vi "Read All Sensor Data.vi"(8 "error in (no error)":errorcluster, 11 "LS218 in":refnum<class "LS218.lvclass">) -> (0 "error out":errorcluster, 3 "LS218 out":refnum<class "LS218.lvclass">)   [LabVIEW 2015, in "LS218.lvlib" / "LS218.lvclass"]
uses:
  LS218.lvclass
  PV-Enum.ctl
  LS218.lvclass/LS218.ctl
  CSPP_Core/Classes/CS++ProcessVariables/PVConnection/PVConnection.lvclass/PVConnection.ctl
  CSPP_Core/Classes/CS++ProcessVariables/ProcessVariable/PV.lvclass/PV.ctl
  CSPP_Core/Classes/CS++ProcessVariables/ProcessVariable/Write Data.vi
  CSPP_Core/Classes/CS++ProcessVariables/ProcessVariable/Write Error.vi
  CSPP_Core/Classes/CS++ProcessVariables/ProcessVariable/Write status.vi
  CSPP_Core/Classes/CS++ProcessVariables/ProcessVariable/Write Quality.vi
  CSPP_Core/Classes/CS++ProcessVariables/ProcessVariable/Write Timestamp.vi
  CSPP_Core/Classes/CS++ProcessVariables/ProcessVariable/PV.lvclass
  <instrlib>/Lake Shore Cryotronics 218/Lake Shore Cryotronics 218.lvlib
  CSPP_Core/Classes/CS++ProcessVariables/PVConnection/PVConnection.lvclass
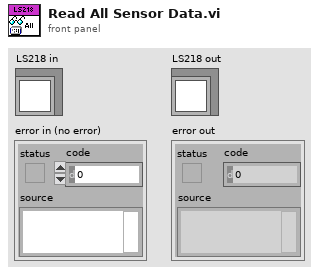
[diagram p1: front panel]
types:
  T1 = typedef "LS218.lvlib/LS218.lvclass/PV-Enum.ctl" = enum16{"T0", "T1", "T2", "T3", "T4", "T5", "T6", "T7", "Relay", "S0", "S1", "S2", "S3", "S4", "S5", "S6", "S7"}
  T2 = cluster{"Relay 1":bool, "Relay  2":bool, "Relay 3":bool, "Relay 4":bool, "Relay 5":bool, "Relay 6":bool, "Relay 7":bool, "Relay 8":bool}
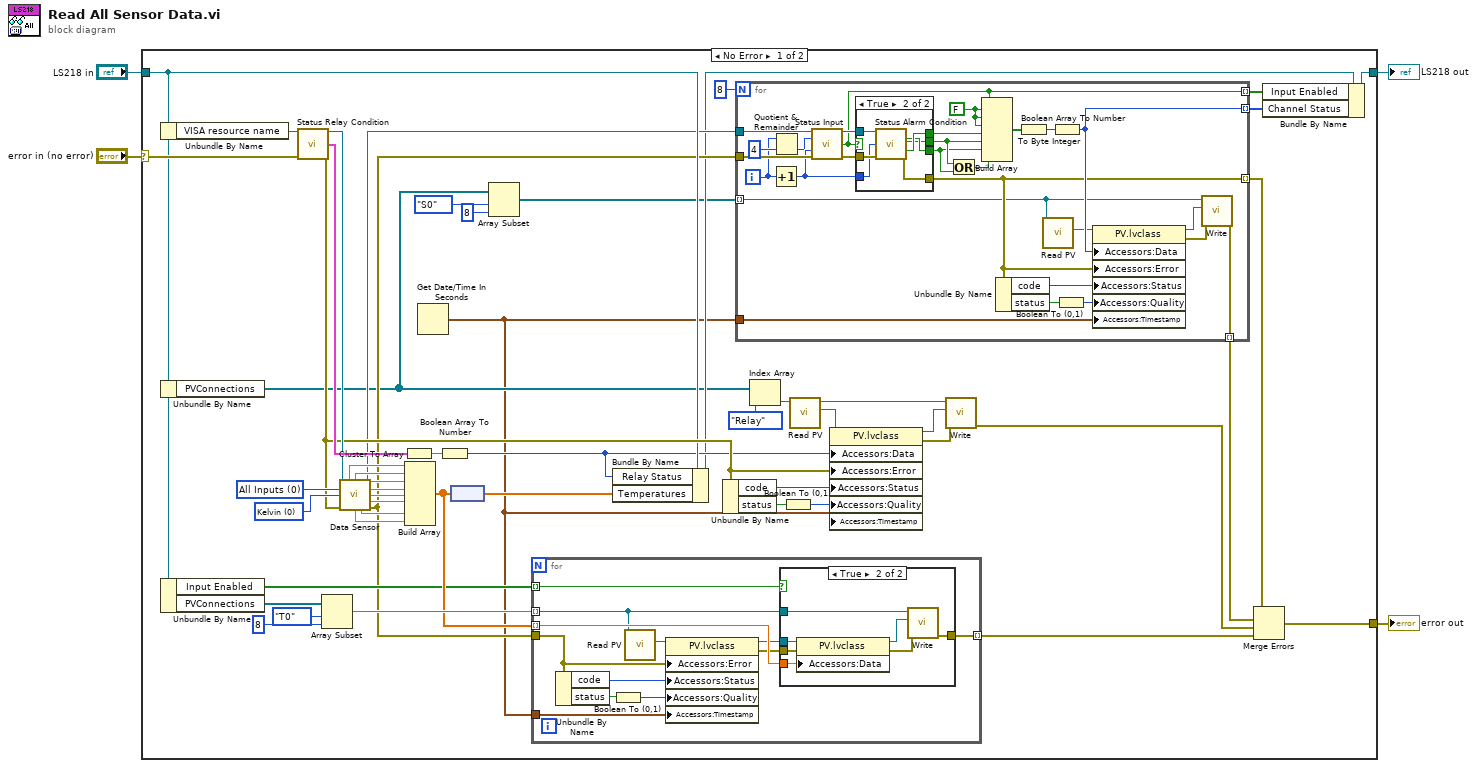
[diagram p0: block diagram]
diagram:
  n1 = case shown="No Error" "error in (no error)" {
    selector: "error in (no error)" -> [w28 w111]
    tunnel: [w40 w111] -> w3
    tunnel: [w17 w110] -> w1
    tunnel: "LS218 in" -> [w26 w110]
    frame No Error {
      w54 = u16 0 items=["All Inputs", "1", "2", "3", "4", "5", "6", "7", "8"] ("Input (0:All)")
      w55 = u16 0 items=["Kelvin", "Celsius", "Sensor Units", "Linear Data"] ("Data Source (0:Kelvin)")
      n2 = Unbundle By Name(w26) -> ("VISA resource name"=w30:refnum<visa-resource-name>)
      n3 = Unbundle By Name(w26) -> ("PVConnections"=w14:refnum<class "PVConnection.lvclass">[])
      n4 = Unbundle By Name(w26) -> ("Input Enabled"=w39:bool[], "PVConnections"=w44:refnum<class "PVConnection.lvclass">[])
      n5 = call <instrlib>:"Status Relay Condition.vi"("VISA resource name"=w30, "error in (no error)"=w28) -> ("VISA resource name out"=w29:refnum<visa-resource-name>, "Relay Status"=w37:T2, "error out"=w27:errorcluster)  [unwired: 11 in]
      n6 = Array Subset(array=w44, index=PV-Enum."T0" ("PV-Enum"), length=8) -> (w42:refnum<class "PVConnection.lvclass">[])
      n7 = call <instrlib>:"Data Sensor.vi"("VISA resource name"=w29, "Input (0:All)"=w54, "Data Source (0:Kelvin)"=w55, "error in (no error)"=w27) -> ("Input 1"=w53:dbl, "Input 2"=w52:dbl, "Input 3"=w51:dbl, "VISA resource name out"=w22:refnum<visa-resource-name>, "Input 4"=w50:dbl, "Input 5"=w49:dbl, "Input 6"=w48:dbl, "Input 8"=w46:dbl, "Input 7"=w47:dbl, "error out"=w21:errorcluster)  [unwired: 2 in]
      n8 = Cluster To Array(cluster=w37) -> (array=w38:bool[])
      n9 = Build Array(w53, w52, w51, w50, w49, w48, w47, w46) -> (w41:dbl[])
      n10 = Get Date/Time In Seconds() -> (seconds since 1Jan1904=w10:timestamp)
      n11 = Boolean Array To Number(Boolean array=w38) -> (number=w25:u32)
      n12 = node(w41) -> (w45:dbl[unit][])
      n13 = Array Subset(array=w14, index=PV-Enum."S0" ("PV-Enum"), length=8) -> (w11:refnum<class "PVConnection.lvclass">[])
      n14 = for {
        tunnel: w42 -> [w57] mode=indexing
        tunnel: w41 -> [w64] mode=indexing
        tunnel: w39 -> [w62] mode=indexing
        tunnel: w10 -> [w58]
        tunnel: w21 -> [w59]
        tunnel: [w60] -> w23 mode=indexing
        n15 = Unbundle By Name(w59) -> ("code"=w67:i32, "status"=w66:bool)
        n16 = Boolean To (0,1)(Boolean=w66) -> (0, 1=w65:i16)
        n17 = call "Read PV.vi"("PVConnection in"=w57) -> ("PV"=w56:refnum<class "PV.lvclass">)  [unwired: 8 in, 2 out]
        n18 = property class="PV.lvclass"(reference=w56, "Accessors:Error"=w59, "Accessors:Status"=w67, "Accessors:Quality"=w65, "Accessors:Timestamp"=w58) -> (reference out=w61:refnum<class "PV.lvclass">, error out=w63:errorcluster)  [unwired: 1 in]
        n19 = case shown="True" w62 {
          tunnel: w57 -> [_ w74]
          tunnel: w61 -> [_ w73]
          tunnel: w64 -> [_ w72]
          tunnel: w63 -> [_ w70]
          tunnel: [_ w68] -> w60
          frame False {
          }
          frame True {
            n20 = property class="PV.lvclass"(reference=w73, error in=w70, "Accessors:Data"=w72) -> (reference out=w71:refnum<class "PV.lvclass">, error out=w69:errorcluster)
            n21 = call "Write.vi"("error in (no error)"=w69, "PV"=w71, "PVConnection in"=w74) -> ("error out"=w68:errorcluster)  [unwired: 7 in, 1 out]
          }
        }
      }
      n22 = Bundle By Name(cluster=w26, "Relay Status"=w25, "Temperatures"=w45) -> (w18:refnum<class "LS218.lvclass">)
      n23 = Unbundle By Name(w27) -> ("code"=w31:i32, "status"=w33:bool)
      n24 = for {
        N: 8 -> [_]
        tunnel: w22 -> [w101]
        tunnel: w21 -> [w98]
        tunnel: [w94] -> w20 mode=indexing
        tunnel: [w79] -> w9 mode=indexing
        tunnel: [w81] -> w12 mode=indexing
        tunnel: w11 -> [w76] mode=indexing
        tunnel: w10 -> [w80]
        tunnel: [w78] -> w8 mode=indexing
        i -> [w96]
        w93 = FALSE
        n25 = Increment(x=w96) -> (x+1=w95:i32)
        n26 = Quotient & Remainder(x=w96, y=4) -> (floor(x/y)=w77:i32)  [unwired: 1 out]
        n27 = call <instrlib>:"Status Input.vi"("VISA resource name"=w101, "Input Group (0:Inputs 1-4)"=w77, "Input (1)"=w95, "error in (no error)"=w98) -> ("VISA resource name out"=w100:refnum<visa-resource-name>, "Input Off/On"=w94:bool, "error out"=w99:errorcluster)  [unwired: 7 in, 2 out]
        n28 = case shown="True" w94 {
          tunnel: w100 -> [_ w109]
          tunnel: w99 -> [w102 w108]
          tunnel: w95 -> [_ w107]
          tunnel: [_ w105] -> w92
          tunnel: [_ w103] -> w91
          tunnel: [_ w104] -> w90
          tunnel: [w102 w106] -> w79
          frame False {
          }
          frame True {
            n29 = call <instrlib>:"Status Alarm Condition.vi"("VISA resource name"=w109, "Input (1)"=w107, "error in (no error)"=w108) -> ("Alarm High Status"=w104:bool, "Alarm Low Status"=w103:bool, "Beeper Status"=w105:bool, "error out"=w106:errorcluster)  [unwired: 8 in, 1 out]
          }
        }
        n30 = Or(x=w91, y=w90) -> (x .or. y?=w89:bool)
        n31 = Build Array(w94, w93, w93, w93, w92, w91, w90, w89) -> (w88:bool[])
        n32 = Unbundle By Name(w79) -> ("code"=w87:i32, "status"=w85:bool)
        n33 = Boolean Array To Number(Boolean array=w88) -> (number=w82:u32)
        n34 = call "Read PV.vi"("PVConnection in"=w76) -> ("PV"=w75:refnum<class "PV.lvclass">)  [unwired: 8 in, 2 out]
        n35 = To Byte Integer(number=w82) -> (8bit integer=w81:i8)
        n36 = Boolean To (0,1)(Boolean=w85) -> (0, 1=w86:i16)
        n37 = property class="PV.lvclass"(reference=w75, "Accessors:Data"=w81, "Accessors:Error"=w79, "Accessors:Status"=w87, "Accessors:Quality"=w86, "Accessors:Timestamp"=w80) -> (reference out=w84:refnum<class "PV.lvclass">, error out=w83:errorcluster)  [unwired: 1 in]
        n38 = call "Write.vi"("error in (no error)"=w83, "PV"=w84, "PVConnection in"=w76) -> ("error out"=w78:errorcluster)  [unwired: 7 in, 1 out]
      }
      n39 = Index Array(array=w14, index=PV-Enum."Relay" ("PV-Enum")) -> (element=w6:refnum<class "PVConnection.lvclass">)
      n40 = Boolean To (0,1)(Boolean=w33) -> (0, 1=w32:i16)
      n41 = call "Read PV.vi"("PVConnection in"=w6) -> ("PV"=w7:refnum<class "PV.lvclass">, "PVConnection out"=w5:refnum<class "PVConnection.lvclass">)  [unwired: 8 in, 1 out]
      n42 = property class="PV.lvclass"(reference=w7, "Accessors:Data"=w25, "Accessors:Error"=w27, "Accessors:Status"=w31, "Accessors:Quality"=w32, "Accessors:Timestamp"=w10) -> (reference out=w35:refnum<class "PV.lvclass">, error out=w36:errorcluster)  [unwired: 1 in]
      n43 = call "Write.vi"("error in (no error)"=w36, "PV"=w35, "PVConnection in"=w5) -> ("error out"=w24:errorcluster)  [unwired: 7 in, 1 out]
      n44 = Merge Errors(w9, w8, w24, w23) -> (w40:errorcluster)
      n45 = Bundle By Name(cluster=w18, "Input Enabled"=w20, "Channel Status"=w12) -> (w17:refnum<class "LS218.lvclass">)
    }
    frame Error {
    }
  }
  "error out" <- w3
  "LS218 out" <- w1
